vi "Read Address.vi"(8 "error in (no error)":errorcluster, 11 "ServerConfig in":refnum<class "ServerConfig.lvclass">) -> (0 "error out":errorcluster, 2 "Address":string="127.0.0.1", 3 "ServerConfig out":refnum<class "ServerConfig.lvclass">)   [LabVIEW 2022 SP3, in "TcpServer.lvlib" / "ServerConfig.lvclass"]
uses:
  ServerConfig.lvclass
  ServerConfig.lvclass/ServerConfig.ctl
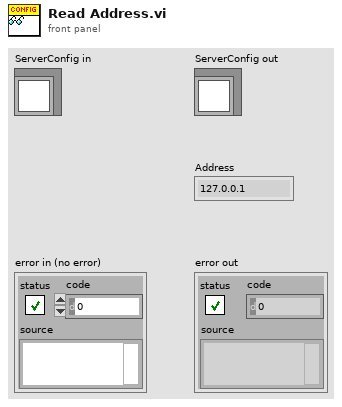
[diagram p1: front panel]
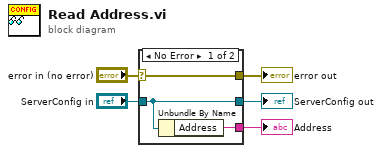
[diagram p0: block diagram]
diagram:
  n1 = case shown="No Error" "error in (no error)" {
    selector: "error in (no error)" -> [w8 w9]
    tunnel: [w8 w9] -> w4
    tunnel: [w7 w10] -> w2
    tunnel: "ServerConfig in" -> [w7 w10]
    tunnel: [w6 _] -> w1
    frame No Error {
      n2 = Unbundle By Name(w7) -> ("Address"=w6:string)
    }
    frame Error {
    }
  }
  "error out" <- w4
  "ServerConfig out" <- w2
  "Address" <- w1
